vi "Transform_GetXY.vi"(11 "inTRANSFORM":T1={"TRANSLATION"={"X"=0.0, "Y"=0.0}, "ROTATION"={"VALUE"=0.0, "COS"=1.0, "SIN"=0.0}}) -> (1 "Y":dbl format="%14.3f", 3 "X":dbl format="%14.3f")   [LabVIEW 2019, in "Trajectory_Library.lvlib"]
doc: "Returns the translation component of the transformation.\n\nParameters:\n - IN TRANSFORM - THis TRANSFORM data structure\n\nReturns:\n - TRANSLATION - The translational component of the transform."
uses:
  TRANSFORM2D.ctl
  TRANSLATION2D.ctl
  ROTATION2D.ctl
  Trajectory_Library.lvlib
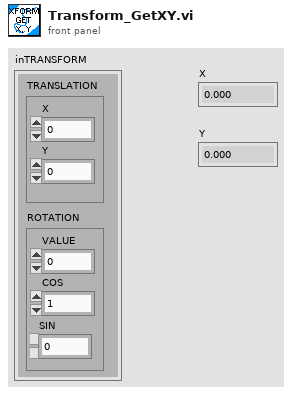
[diagram p1: front panel]
types:
  T1 = typedef "Trajectory_Library.lvlib/TRANSFORM2D.ctl" = cluster{"TRANSLATION":T2, "ROTATION":T3}
  T2 = typedef "Trajectory_Library.lvlib/TRANSLATION2D.ctl" = cluster{"X":dbl, "Y":dbl}
  T3 = typedef "Trajectory_Library.lvlib/ROTATION2D.ctl" = cluster{"VALUE":dbl, "COS":dbl, "SIN":dbl}
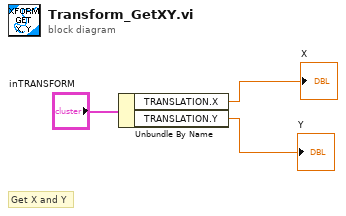
[diagram p0: block diagram]
diagram:
  # "Get X and Y"
  n1 = Unbundle By Name("inTRANSFORM") -> ("TRANSLATION.X"=→"X":dbl, "TRANSLATION.Y"=→"Y":dbl)
